vi "Execute.vi"(8 "error in":errorcluster, 10 "Change Laser Modulation in":refnum<class "Change Laser Modulation.lvclass">, 11 "Object In":refnum<class>) -> (0 "error out":errorcluster, 3 "Object Out":refnum<class>)   [LabVIEW 2014, in "Change Laser Modulation.lvclass"]
doc: "Abstract method for accomplishing the execution of a command directed to an instrument object on the wire."
uses:
  Change Laser Modulation.lvclass
  FPGA/Session/Exscalabar FPGA.lvclass
  Instrument/ePAS.lvclass
  Instrument/ePAS.lvclass/ePAS.ctl
  reusable/Instrument/Instrument.lvclass/Instrument.ctl
  Instrument/Accessors/Read FPGA Session.vi
  reusable/Instrument/Read Log Session.vi
  FPGA/Session/Read Ex FPGA Ref.vi
  <userlib>/_Session Fwk/Session - Root.lvclass
  reusable/Session APIs/Session Log/System Log.lvclass
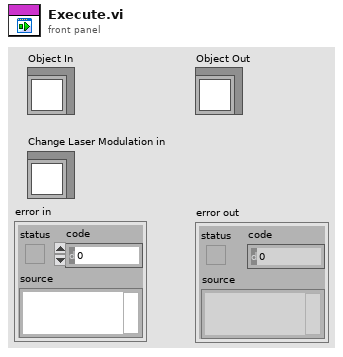
[diagram p1: front panel]
types:
  T1 = typedef "Session - Root.lvclass/Session Handle.ctl" = refnum<data-value>
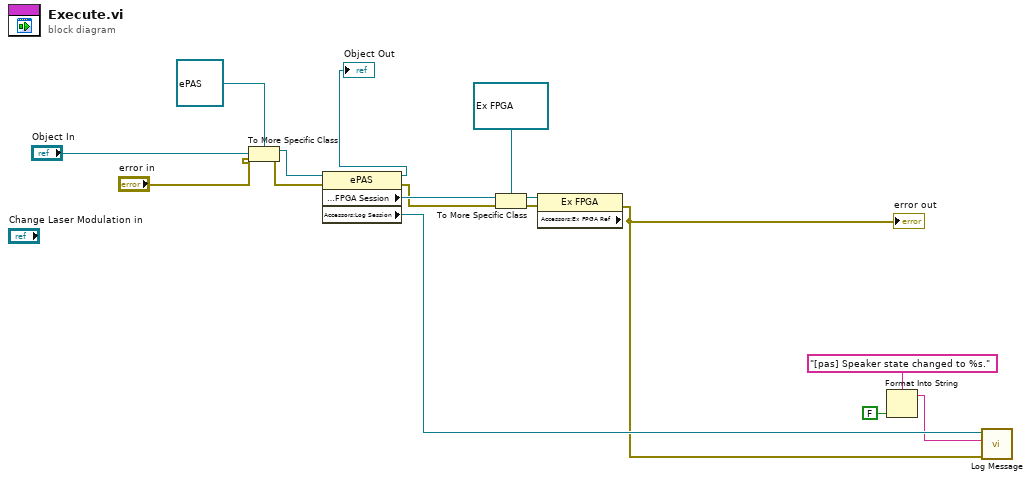
[diagram p0: block diagram]
diagram:
  n1 = To More Specific Class(target class=refnum<class "ePAS.lvclass"> refnum ("ePAS.lvclass"), reference="Object In", error in="error in") -> (specific class reference=w4:refnum<class "ePAS.lvclass">, error out=w3:errorcluster)
  n2 = property class="ePAS"(reference=w4, error in=w3) -> (reference out=→"Object Out":refnum<class "ePAS.lvclass">, error out=w8:errorcluster, "Accessors:FPGA Session"=w13:T1, "Accessors:Log Session"=w12:T1)
  n3 = To More Specific Class(target class=refnum<data-value> refnum ("Session Handle"), reference=w13, error in=w8) -> (specific class reference=w15:refnum<data-value>, error out=w14:errorcluster)
  n4 = property class="Ex FPGA" props=["Accessors:Ex FPGA Ref"](reference=w15, error in=w14) -> (error out=w9:errorcluster)  [unwired: 2 out]
  "error out" <- w9
  n5 = Format Into String(format string="[pas] Speaker state changed to %s.", FALSE ("input 1")) -> (resulting string=w10:string)  [unwired: 2 in, 1 out]
  n6 = call "Log Message.vi"("error in"=w9, "MSG In"=w10, "session in"=w12) -> ()  [unwired: 7 in, 2 out]
